vi "Step Association Delete Instrument.vi"(8 "error in (no error)":errorcluster, 10 "iInstrument (0)":i32, 11 "Connection Refnum":T1) -> (0 "error out":errorcluster, 3 "Connection Refnum":T1)   [LabVIEW 2011]
uses:
  Summitek EXT/ODBC/SQL Controls/Connection Refnum.ctl
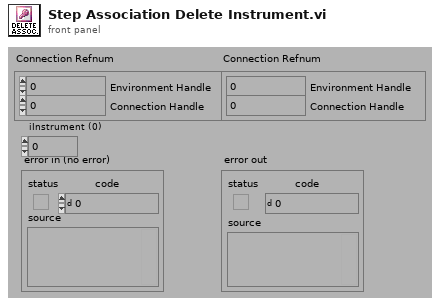
[diagram p1: front panel]
types:
  T1 = typedef "Connection Refnum.ctl" = cluster{"Environment Handle":i32, "Connection Handle":i32}
  T2 = typedef "Statement Refnum.ctl" = cluster{"Statement Handle":i32, "Parameter Number":u16}
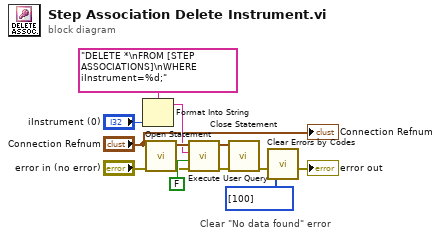
[diagram p0: block diagram]
diagram:
  # "Clear \"No data found\" error"
  n1 = Format Into String(format string="DELETE *\nFROM [STEP ASSOCIATIONS]\nWHERE iInstrument=%d;" ("User Query"), "iInstrument (0)") -> (resulting string=w8:string)  [unwired: 2 in, 1 out]
  n2 = call "Open Statement.vi"("error in (no error)"="error in (no error)", "Connection Refnum"="Connection Refnum") -> ("error out"=w10:errorcluster, "Statement Refnum"=w9:T2)  [unwired: 4 out]
  n3 = call "Execute User Query.vi"("error in (no error)"=w10, "Return Data? (f)"=FALSE, "User Query"=w8, "Statement Refnum"=w9) -> ("error out"=w11:errorcluster, "Statement Refnum"=w12:T2)  [unwired: 2 out]
  n4 = call "Close Statement.vi"("error in (no error)"=w11, "Statement Refnum"=w12) -> ("error out"=w4:errorcluster)  [unwired: 5 out]
  n5 = call "Clear Errors by Codes.vi"("Error Codes\nto Clear (Empty)"=i32[] [100] ("Error Codes\nto Clear (Empty)"), "error in (no error)"=w4) -> ("error out"=→"error out":errorcluster)  [unwired: 5 out]
  "Connection Refnum" <- "Connection Refnum"
